vi "Lab2_demodulation.vi"() -> ()   [LabVIEW 2010]
uses:
  <vilib>/measure/maspectr.llb/FFT Spectrum (Mag-Phase) for N Chan.vi
  <vilib>/measure/NI_MABase.lvlib
  <vilib>/measure/NI_MAPro.lvlib
  <vilib>/ptbypt/NI_PtbyPt.lvlib
panel:
  out "DC estimate (V)":dbl format="%0.2f"
  out "Baseband/DSB":dbl
  out "Demod DSB/AM DSB-SC":dbl
  out "Demod DSB-SC/AM DSB-SC":dbl
  out "Demodulated DSB (time)":dynamicdata(graph) caption="Filtered Signal"
  out "Demodulated DSB (frequency)":cluster{"f0":dbl, "df":dbl, "magnitude":dbl[]}[](graph) caption="Filtered Signal"
  out "Baseband Signal (frequency)":cluster{"f0":dbl, "df":dbl, "magnitude":dbl[]}(graph)
  out "Demodulated DSB-SC (frequency)":cluster{"f0":dbl, "df":dbl, "magnitude":dbl[]}[](graph) caption="Filtered Signal"
  out "Demodulated DSB-SC (time)":dynamicdata(graph) caption="Filtered Signal"
  in  "stop":bool
  out "Baseband Signal (time)":waveform(dbl)(graph)
  in  "mod index":dbl(slide)=1.0 scale=0.0..1.0
  in  "modulation frequency":dbl(knob)=10.0 scale=0.0..1000.0
  in  "carrier frequency":dbl(knob)=10.0 scale=0.0..500000.0
  in  "carrier amplitude":dbl(slide) scale=0.0..1.0
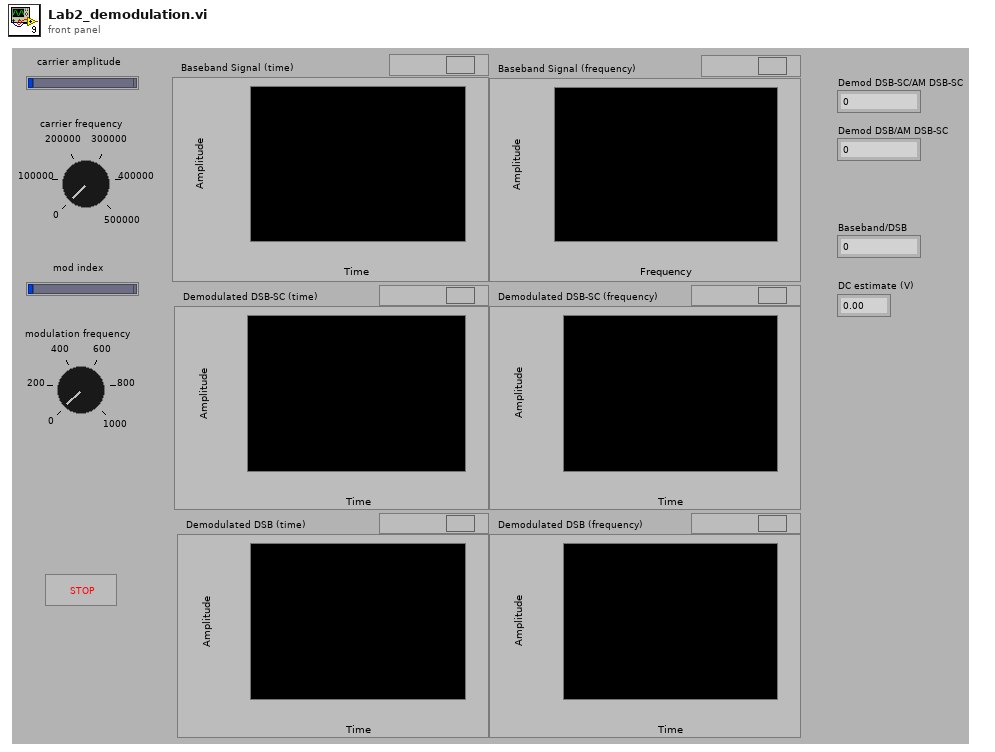
[diagram p1: front panel]
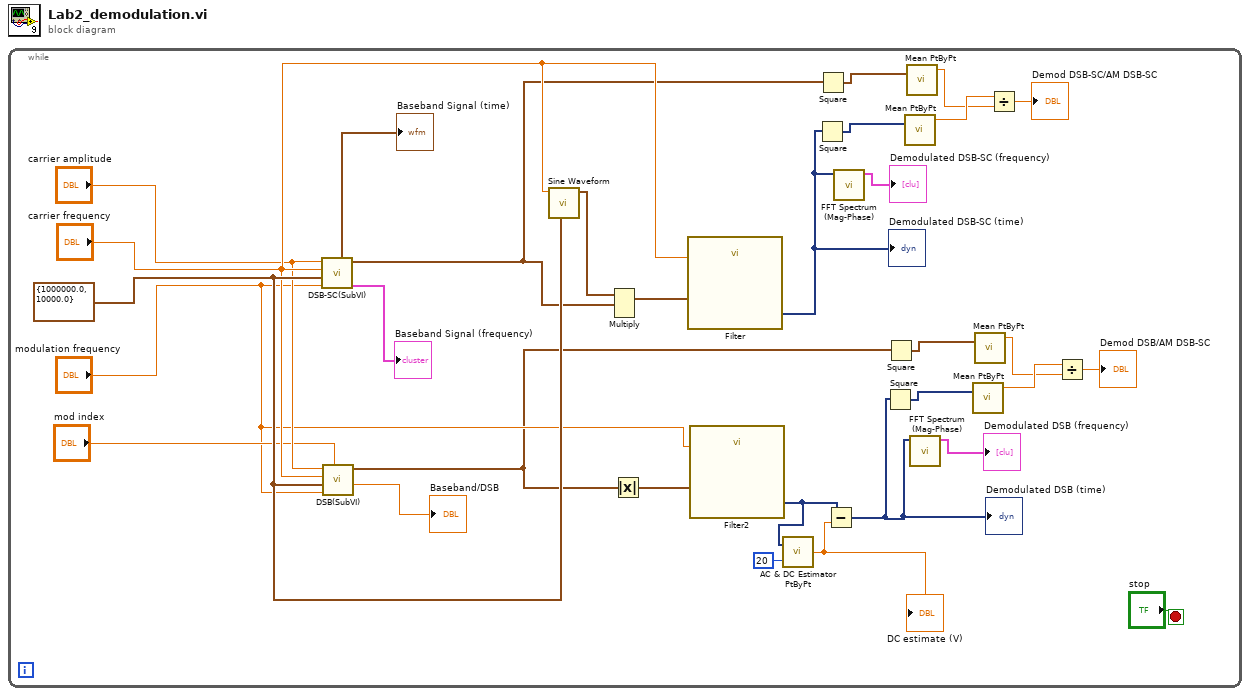
[diagram p0: block diagram]
diagram:
  n1 = while {
    stop <- "stop" stop-if-true
    w30 = cluster{"Fs":dbl, "#s":dbl} {"Fs"=1000000.0, "#s"=10000.0} ("sampling info")
    n2 = call "DSB-SC(SubVI).vi"("modulation frequency"="modulation frequency", "sampling info"=w30, "carrier frequency"="carrier frequency", "carrier amplitude"="carrier amplitude") -> ("baseband signal (frequency-domain)"=→"Baseband Signal (frequency)":cluster{"f0":dbl, "df":dbl, "magnitude":dbl[]}, "modulated signal (time-domain)"=w8:waveform(dbl), "baseband signal (time-domain)"=→"Baseband Signal (time)":waveform(dbl))  [unwired: 1 in, 2 out]
    n3 = call "DSB(SubVI).vi"("mod index"="mod index", "modulation frequency"="modulation frequency", "sampling info"=w30, "carrier frequency"="carrier frequency", "carrier amplitude"="carrier amplitude") -> ("power ratio"=→"Baseband/DSB":dbl, "modulated signal (time-domain)"=w5:waveform(dbl))  [unwired: 3 out]
    n4 = call <vilib>:"Sine Waveform.vi"("sampling info"=w30, "frequency"="carrier frequency") -> ("signal out"=w4:waveform(dbl))  [unwired: 8 in, 1 out]
    n5 = Multiply(1:w8, 2:w4) -> (0:w29:waveform(dbl))  [unwired: 1 in, 1 out]
    n6 = Absolute Value(x=w5) -> (abs(x)=w6:waveform(dbl))
    n7 = call "Filter"("Lower Cut-Off"="carrier frequency", "Signal"=w29) -> ("Filtered Signal"=w13:dynamicdata)  [unwired: 8 in, 1 out]
    "Demodulated DSB-SC (time)" <- w13
    n8 = call "Filter2"("Lower Cut-Off"="modulation frequency", "Signal"=w6) -> ("Filtered Signal"=w3:dynamicdata)  [unwired: 8 in, 1 out]
    n9 = call <vilib>:"AC & DC Estimator PtByPt.vi"("signal"=w3, "sample length"=20) -> ("DC estimate (V)"=w2:dbl)  [unwired: 1 in, 2 out]
    "DC estimate (V)" <- w2
    n10 = Square(x=w13) -> (x^2=w23:dynamicdata)
    n11 = Square(x=w8) -> (x^2=w22:waveform(dbl))
    n12 = Subtract(x=w3, y=w2) -> (x-y=w11:dynamicdata)
    "Demodulated DSB (time)" <- w11
    n13 = call-poly <vilib>:"FFT Spectrum (Mag-Phase).vi"("time signals"=w13) -> ("magnitudes"=→"Demodulated DSB-SC (frequency)":cluster{"f0":dbl, "df":dbl, "magnitude":dbl[]}[])  [unwired: 6 in, 4 out]
    n14 = Square(x=w11) -> (x^2=w18:dynamicdata)
    n15 = Square(x=w5) -> (x^2=w17:waveform(dbl))
    n16 = call <vilib>:"Mean PtByPt.vi"("x"=w23) -> ("mean"=w20:dbl)  [unwired: 3 in, 1 out]
    n17 = call <vilib>:"Mean PtByPt.vi"("x"=w22) -> ("mean"=w19:dbl)  [unwired: 3 in, 1 out]
    n18 = call-poly <vilib>:"FFT Spectrum (Mag-Phase).vi"("time signals"=w11) -> ("magnitudes"=→"Demodulated DSB (frequency)":cluster{"f0":dbl, "df":dbl, "magnitude":dbl[]}[])  [unwired: 6 in, 4 out]
    n19 = call <vilib>:"Mean PtByPt.vi"("x"=w18) -> ("mean"=w15:dbl)  [unwired: 3 in, 1 out]
    n20 = call <vilib>:"Mean PtByPt.vi"("x"=w17) -> ("mean"=w14:dbl)  [unwired: 3 in, 1 out]
    n21 = Divide(x=w20, y=w19) -> (x/y=→"Demod DSB-SC/AM DSB-SC":dbl)
    n22 = Divide(x=w15, y=w14) -> (x/y=→"Demod DSB/AM DSB-SC":dbl)
  }
